vi "Write UserEvent Ref.vi"(8 "error in (no error)":errorcluster, 10 "UserEvent Ref":refnum<user-event>, 11 "UserEventMessageTransport":refnum<class "UserEventMessageTransport.lvclass">) -> (0 "error out":errorcluster, 3 "UserEventMessageTransport":refnum<class "UserEventMessageTransport.lvclass">)   [LabVIEW 2016, in "UserEventMessageTransport.lvclass"]
uses:
  UserEventMessageTransport.lvclass
  IMessagePayload/IMessagePayload.lvclass
  UserEventMessageTransport.lvclass/UserEventMessageTransport.ctl
panel:
  # "INPUTS"
  # "OUTPUTS"
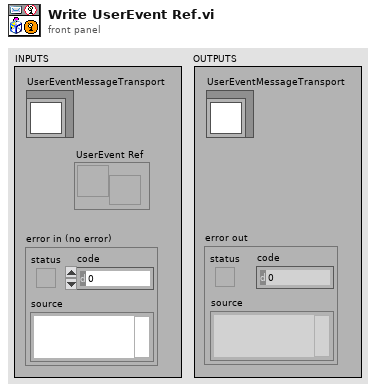
[diagram p1: front panel]
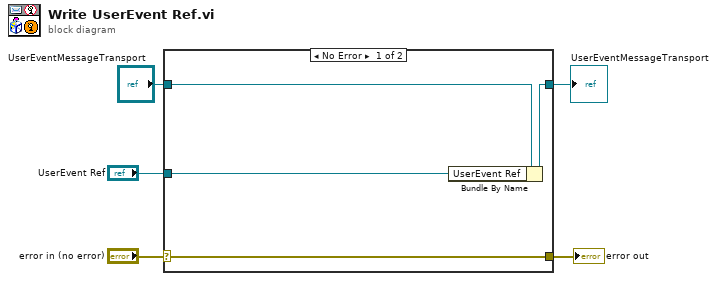
[diagram p0: block diagram]
diagram:
  n1 = case shown="No Error" "error in (no error)" {
    selector: "error in (no error)" -> [w9 w10]
    tunnel: [w9 w10] -> w4
    tunnel: [w7 w11] -> w2
    tunnel: "UserEventMessageTransport" -> [w8 w11]
    tunnel: "UserEvent Ref" -> [w6 _]
    frame No Error {
      n2 = Bundle By Name(cluster=w8, "UserEvent Ref"=w6) -> (w7:refnum<class "UserEventMessageTransport.lvclass">)
    }
    frame Error {
    }
  }
  "error out" <- w4
  "UserEventMessageTransport" <- w2
